vi "LJstreamUD globals.vi"() -> ()   [LabVIEW 2022 SP3]
panel:
  in  "Graph?":bool[](array[boolean])=[FALSE, FALSE, FALSE, FALSE, FALSE, FALSE, FALSE, FALSE, FALSE, FALSE, FALSE, FALSE, FALSE, FALSE, FALSE, FALSE]
  in  "Graph Buffer":dbl[][](array[numeric]) format="%.3f"
  in  "Working Directory":path
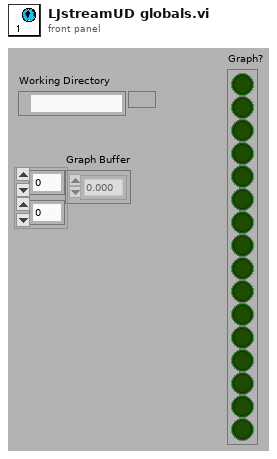
[diagram p1: front panel]
diagram:
